vi "C2.vi"(8 "error in (no error)":errorcluster, 11 "KNR in":T2) -> (0 "error out":errorcluster, 3 "KNR out":T2, 4 "DC Position Offset":i32)   [LabVIEW 2013]
uses:
  <userlib>/KNR OS 3.0 LabVIEW Toolkit/Type Definition/KNR3 Reference.ctl
  <userlib>/_FPGA Interface Advanced Tools/FPGA Interface Base/FPGA Interface Base.lvclass
  <userlib>/KNR OS 3.0 LabVIEW Toolkit/Type Definition/Resource.ctl
  Global 1.vi
panel:
  out "处理前":T1(plugin-control)
  out "最右边的坐标":dbl[][](array[numeric])
  out "处理后":T1(plugin-control)
  out "Error(deg)":ext
  in  "STOP":bool
  out "CM":dbl
  out "e pix":dbl
  out "Aim":dbl
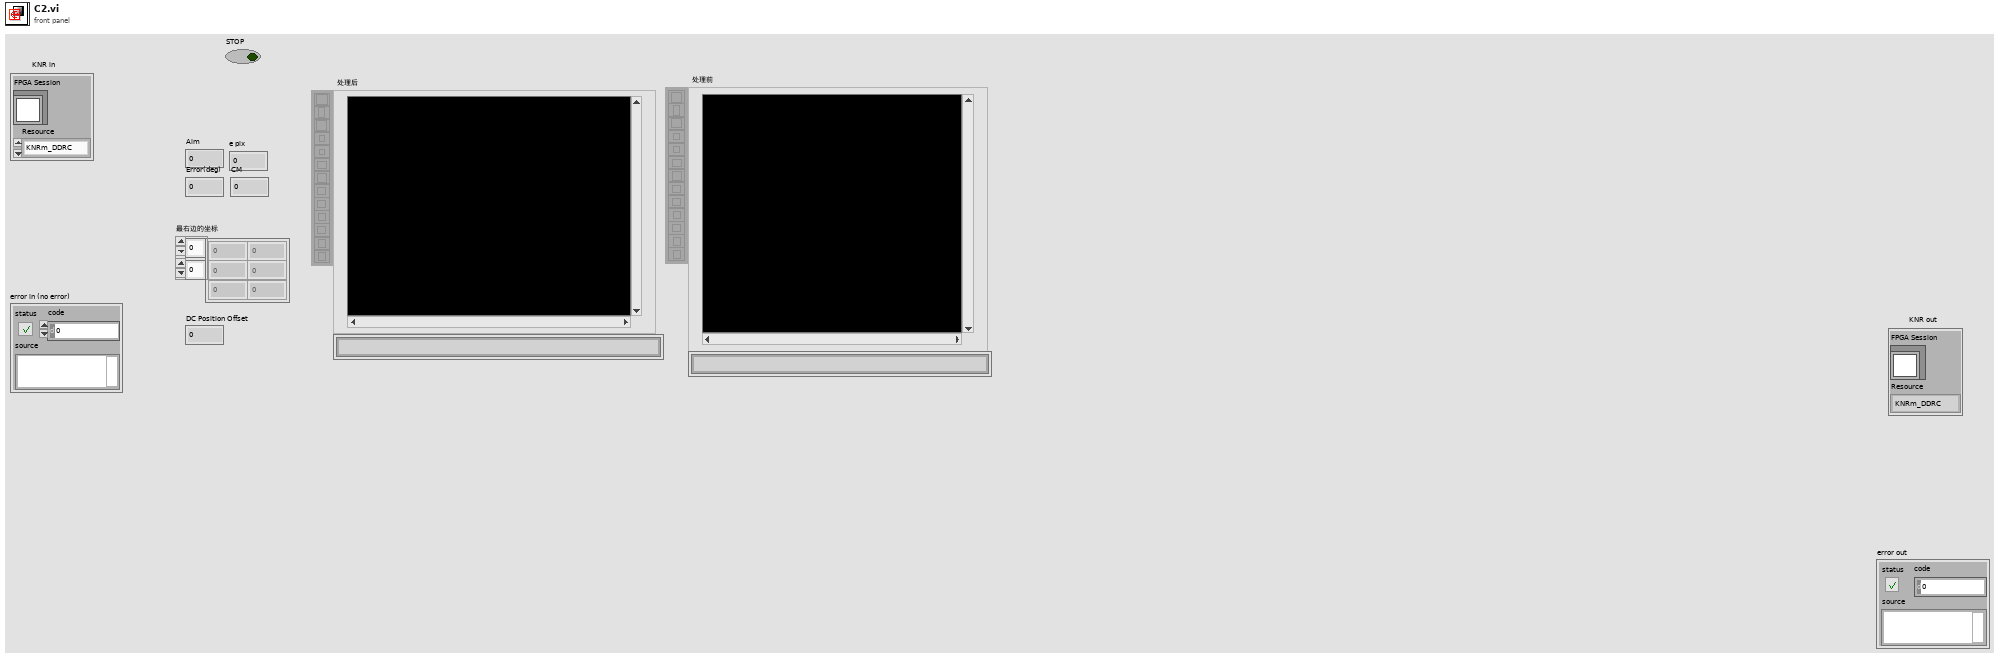
[diagram p1: front panel]
types:
  T1 = typedef "IMAQ Image.ctl" = refnum<image>
  T2 = typedef "KNR3 Reference.ctl" = cluster{"FPGA Session":refnum<class "FPGA Interface Base.lvclass">, "Resource":T3}
  T3 = typedef "Resource.ctl" = enum16{"KNRm_DDRC", "KNRm_DDDD", "KNRm_DDDR", "KNRm_DDDC", "KNR"}
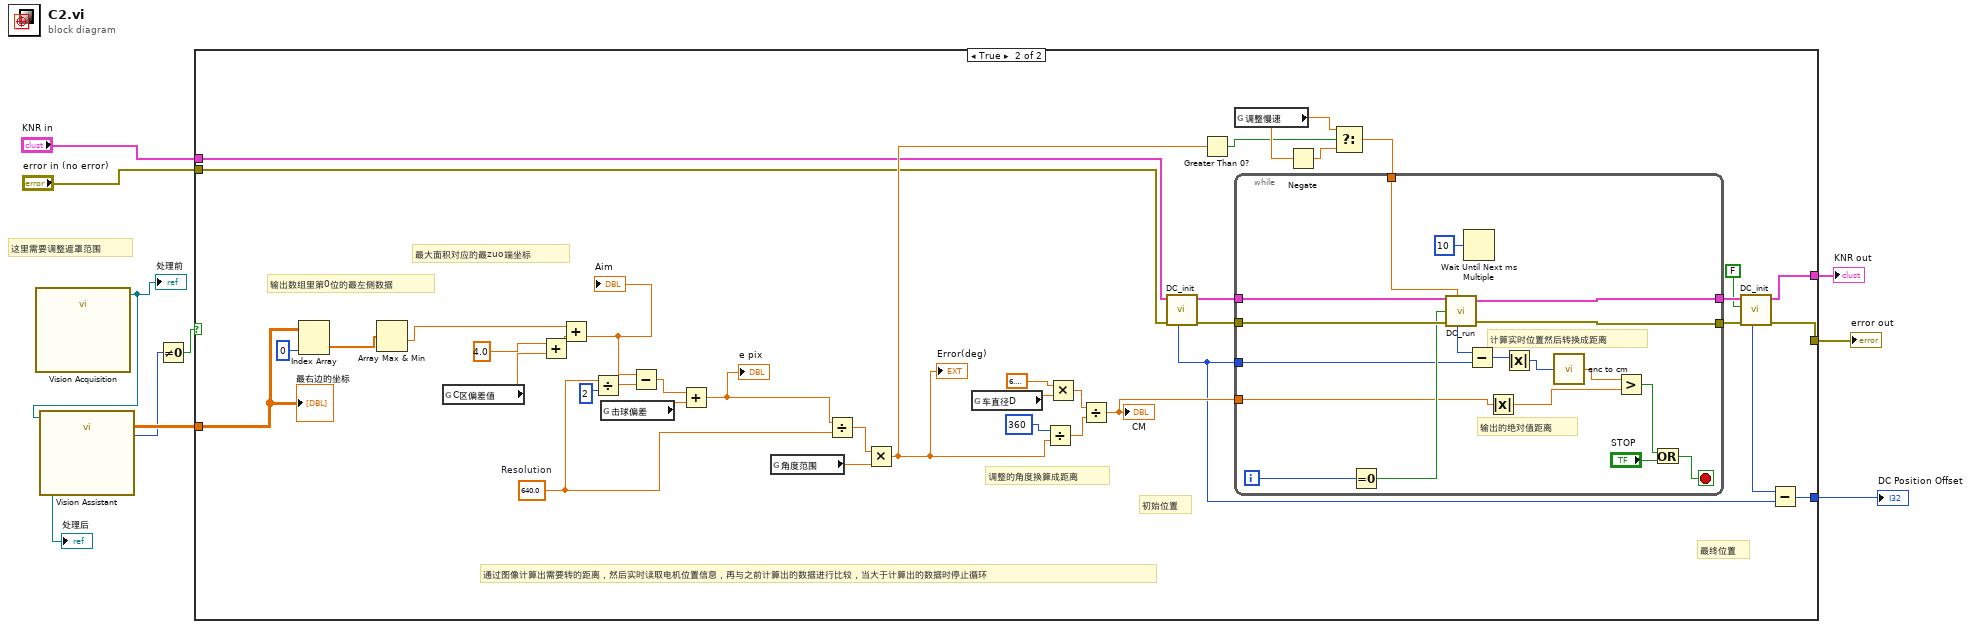
[diagram p0: block diagram]
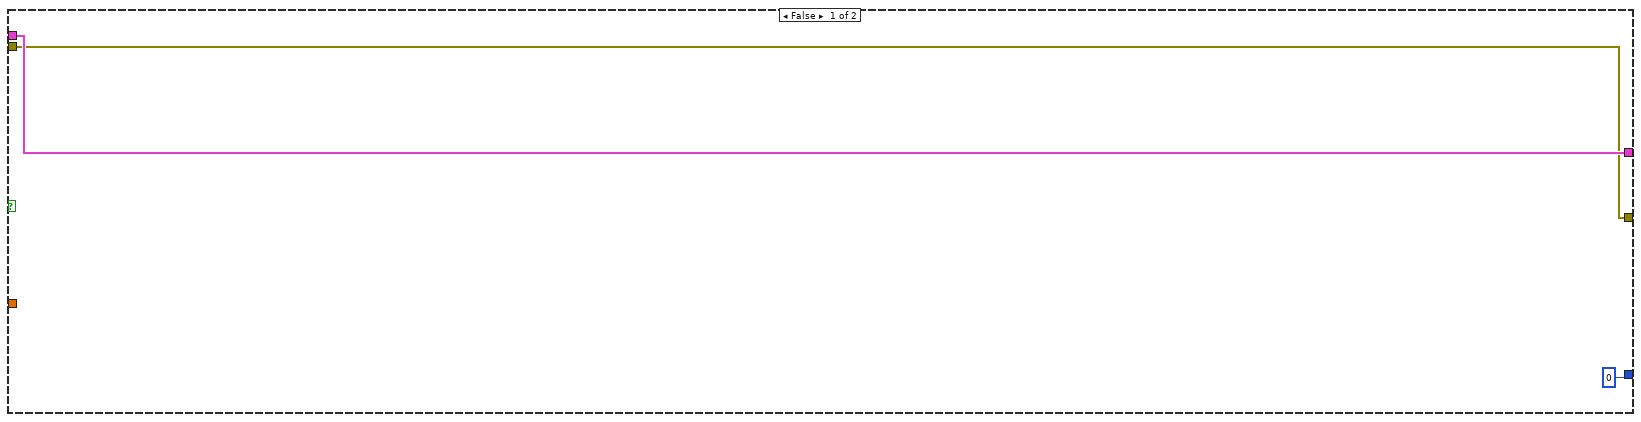
[diagram p2: hidden frame]
diagram:
  # "这里需要调整遮罩范围"
  n1 = call "Vision Acquisition"() -> ("Image Out"=w1:T1)  [unwired: 26 in, 1 out]
  "处理前" <- w1
  n2 = call "Vision Assistant"("Image In"=w1) -> ("Image Out"=→"处理后":T1, "Particle Measurements (Pixels) (Particle Analysis 1)"=w7:dbl[][], "Number of Particles (Particle Analysis 1)"=w4:i32)  [unwired: 23 in, 1 out]
  n3 = Not Equal To 0?(x=w4) -> (x != 0?=w5:bool)
  n4 = case shown="True" w5 {
    tunnel: [w13 w26] -> w10
    tunnel: [w12 w25] -> w9
    tunnel: w7 -> [_ w23]
    tunnel: [0 w22] -> w6
    tunnel: "KNR in" -> [w13 w21]
    tunnel: "error in (no error)" -> [w12 w20]
    frame False {
    }
    frame True {
      w36 = 640.0  # Resolution
      # "最终位置"
      # "最大面积对应的最zuo端坐标"
      # "输出数组里第0位的最左侧数据"
      # "调整的角度换算成距离"
      # "初始位置"
      # "通过图像计算出需要转的距离，然后实时读取电机位置信息，再与之前计算出的数据进行比较，当大于计算出的数据时停止循环"
      n5 = Index Array(array=w23, index (col)=0 ("disabled index (col)")) -> (element=w18:dbl[])  [unwired: 1 in]
      n6 = Array Max & Min(array=w18) -> (min value=w16:dbl)  [unwired: 3 out]
      n7 = global read "Global 1.vi" "C区偏差值"() -> (w17:dbl)
      n8 = Add(x=4.0, y=w17) -> (x+y=w15:dbl)
      n9 = Add(x=w16, y=w15) -> (x+y=w19:dbl)
      "Aim" <- w19
      n10 = Divide(x=w36, y=2) -> (x/y=w35:dbl)
      n11 = global read "Global 1.vi" "击球偏差"() -> (w51:dbl)
      n12 = Subtract(x=w19, y=w35) -> (x-y=w52:dbl)
      n13 = Add(x=w52, y=w51) -> (x+y=w48:dbl)
      "e pix" <- w48
      n14 = global read "Global 1.vi" "角度范围"() -> (w50:dbl)
      n15 = Divide(x=w48, y=w36) -> (x/y=w49:dbl)
      n16 = Multiply(x=w49, y=w50) -> (x*y=w29:dbl)
      "Error(deg)" <- w29
      n17 = global read "Global 1.vi" "车直径D"() -> (w45:dbl)
      n18 = Divide(x=360, y=w29) -> (x/y=w43:dbl)
      n19 = Multiply(x=6.283185307179586, y=w45) -> (x*y=w44:dbl)
      n20 = Divide(x=w44, y=w43) -> (x/y=w40:dbl)
      "CM" <- w40
      n21 = call "DC_init.vi"("error in (no error)"=w20, "KNR in"=w21) -> ("error out"=w41:errorcluster, "KNR out"=w42:T2, "output\nPosition_1"=w33:i32)  [unwired: 6 in, 1 out]
      n22 = Greater Than 0?(x=w29) -> (x > 0?=w30:bool)
      n23 = global read "Global 1.vi" "调整慢速"() -> (w31:dbl)
      n24 = Negate(x=w31) -> (-x=w32:dbl)
      n25 = Select(t=w31, s=w30, f=w32) -> (s? t:f=w28:dbl)
      n26 = while {
        tunnel: w42 -> [w70]
        tunnel: w41 -> [w69]
        tunnel: [w68] -> w39
        tunnel: [w67] -> w38
        tunnel: w40 -> [w58]
        tunnel: w33 -> [w55]
        tunnel: w28 -> [w53]
        i -> [w61]
        stop <- w64 stop-if-true
        # "输出的绝对值距离"
        # "计算实时位置然后转换成距离"
        n27 = Equal To 0?(x=w61) -> (x = 0?=w60:bool)
        n28 = call "DC_run.vi"("KNR in"=w70, "speed_1"=w53, "reinitialize? (F)"=w60, "error in (no error)"=w69) -> ("Position_1"=w54:i32, "KNR out"=w68:T2, "error out"=w67:errorcluster)  [unwired: 2 in, 1 out]
        n29 = Wait Until Next ms Multiple(millisecond multiple=u32 10) -> ()  [unwired: 1 out]
        n30 = Subtract(x=w54, y=w55) -> (x-y=w66:i32)
        n31 = Absolute Value(x=w58) -> (abs(x)=w65:dbl)
        n32 = Absolute Value(x=w66) -> (abs(x)=w57:i32)
        n33 = call "enc to cm.vi"("E"=w57) -> ("CM"=w56:dbl)  [unwired: 1 in]
        n34 = Greater?(x=w56, y=w65) -> (0:w63:bool)
        n35 = Or(x=w63, y="STOP") -> (x .or. y?=w64:bool)
      }
      n36 = call "DC_init.vi"("error in (no error)"=w38, "Enable Motor(T)"=FALSE, "KNR in"=w39) -> ("error out"=w25:errorcluster, "KNR out"=w26:T2, "output\nPosition_1"=w27:i32)  [unwired: 5 in, 1 out]
      n37 = Subtract(x=w27, y=w33) -> (x-y=w22:i32)
      "最右边的坐标" <- w23
    }
  }
  "error out" <- w9
  "KNR out" <- w10
  "DC Position Offset" <- w6
